vi "Read Signal Quality Statistics.vi"(8 "error in (no error)":errorcluster, 11 "DROPBEAR_Model_Updating in":refnum<class "DROPBEAR_Model_Updating.lvclass">) -> (0 "error out":errorcluster, 2 "Signal Quality Statistics":T1, 3 "DROPBEAR_Model_Updating out":refnum<class "DROPBEAR_Model_Updating.lvclass">)   [LabVIEW 2021, in "DROPBEAR_Model_Updating.lvclass"]
uses:
  DROPBEAR_Model_Updating.lvclass
  Online_SNR/Online_SNR.lvclass
  Online_TRAC/Online_TRAC.lvclass
  Online_Statistic/Online_Statistic.lvclass
  DROPBEAR_Model_Updating.lvclass/DROPBEAR_Model_Updating.ctl
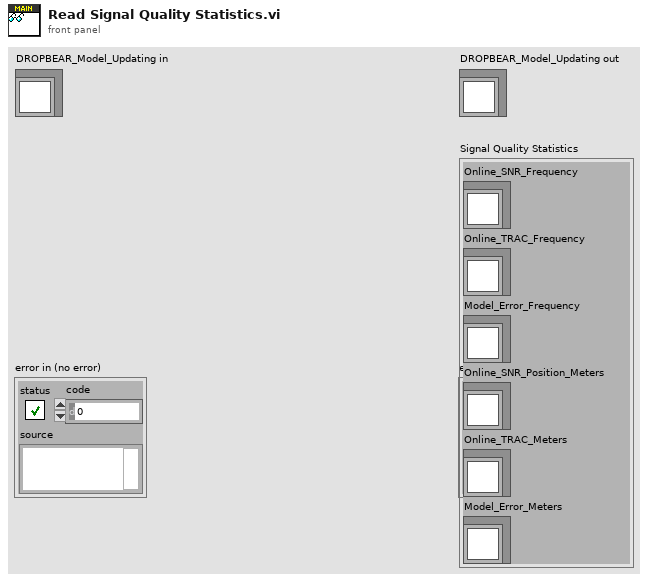
[diagram p1: front panel]
types:
  T1 = cluster{"Online_SNR_Frequency":refnum<class "Online_SNR.lvclass">, "Online_TRAC_Frequency":refnum<class "Online_TRAC.lvclass">, "Model_Error_Frequency":refnum<class "Online_Statistic.lvclass">, "Online_SNR_Position_Meters":refnum<class "Online_SNR.lvclass">, "Online_TRAC_Meters":refnum<class "Online_TRAC.lvclass">, "Model_Error_Meters":refnum<class "Online_Statistic.lvclass">}
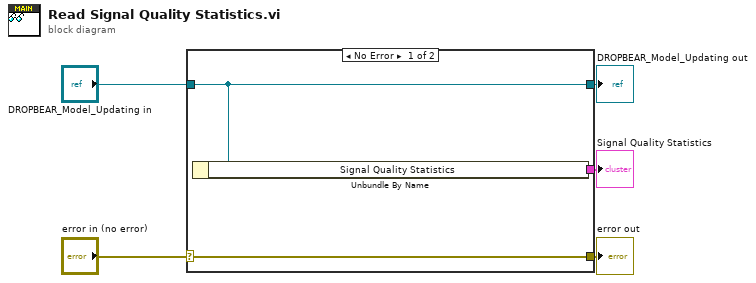
[diagram p0: block diagram]
diagram:
  n1 = case shown="No Error" "error in (no error)" {
    selector: "error in (no error)" -> [w8 w9]
    tunnel: [w8 w9] -> w4
    tunnel: [w7 w10] -> w2
    tunnel: "DROPBEAR_Model_Updating in" -> [w7 w10]
    tunnel: [w6 _] -> w1
    frame No Error {
      n2 = Unbundle By Name(w7) -> ("Signal Quality Statistics"=w6:T1)
    }
    frame Error {
    }
  }
  "error out" <- w4
  "DROPBEAR_Model_Updating out" <- w2
  "Signal Quality Statistics" <- w1
